vi "Process Data.vi"(7 "AdasLvTemplate in":refnum<class "AdasLvTemplate.lvclass">, 8 "error in":errorcluster, 11 "Node in":refnum<class "BLS Chiller Template.lvclass">) -> (0 "error out":errorcluster, 3 "Node out":refnum<class "BLS Chiller Template.lvclass">, 5 "AdasLvTemplate out":refnum<class "AdasLvTemplate.lvclass">)   [LabVIEW 2023, in "BLS Chiller Template.lvlib" / "BLS Chiller Template.lvclass"]
uses:
  BLS Chiller Template.lvclass
  <vilib>/ADAS Replay HIL/ADAS Plugin Utilities/AdasLvTemplate/AdasLvTemplate.lvclass
  BLS Chiller Template.lvclass/BLS Chiller Template.ctl
  bls-capabilities/src/Capabilities/High Level Capabilities/Chiller/Error Channels Write Array.vi
  bls-capabilities/src/Capabilities/High Level Capabilities/Chiller/Temperature Min Read Array.vi
  bls-capabilities/src/Capabilities/High Level Capabilities/Chiller/Temperature Max Read Array.vi
  bls-capabilities/src/Capabilities/High Level Capabilities/Chiller/Temperature Grad Read Array.vi
  bls-capabilities/src/Capabilities/High Level Capabilities/Chiller/Temperature Read Array.vi
  bls-capabilities/src/Capabilities/High Level Capabilities/Chiller/Pressure Min Read Array.vi
  bls-capabilities/src/Capabilities/High Level Capabilities/Chiller/Pressure Max Read Array.vi
  bls-capabilities/src/Capabilities/High Level Capabilities/Chiller/Pressure Grad Read Array.vi
  bls-capabilities/src/Capabilities/High Level Capabilities/Chiller/Pressure Read Array.vi
  bls-capabilities/src/Capabilities/High Level Capabilities/Chiller/Flow Max Read Array.vi
  bls-capabilities/src/Capabilities/High Level Capabilities/Chiller/Flow Min Read Array.vi
  bls-capabilities/src/Capabilities/High Level Capabilities/Chiller/Flow Read Array.vi
  bls-capabilities/src/Capabilities/High Level Capabilities/Chiller/Flow Grad Read Array.vi
  bls-capabilities/src/Capabilities/High Level Capabilities/Chiller/Temperature Write Array.vi
  bls-capabilities/src/Capabilities/High Level Capabilities/Chiller/Pressure Write Array.vi
  bls-capabilities/src/Capabilities/High Level Capabilities/Chiller/Flow Write Array.vi
  bls-capabilities/src/Capabilities/High Level Capabilities/Chiller/Chiller.lvclass
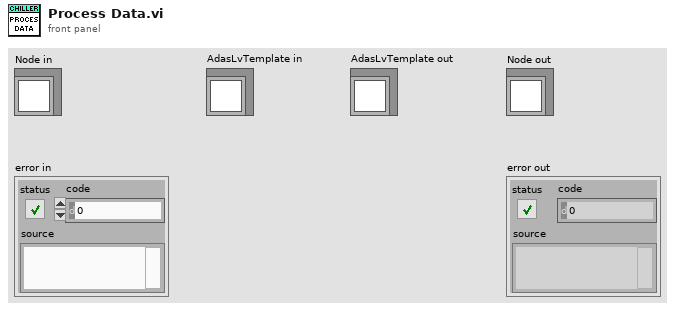
[diagram p1: front panel]
types:
  T1 = typedef "BLS Chiller Template.lvlib/BLS Chiller Template.lvclass/Configuration Params.ctl" = cluster{"Common":T2, "Amount of Channels":u32, "Address":string}
  T2 = typedef "Template Node.lvlib/Template Node.lvclass/Common Configuration Params.ctl" = cluster{"Iteration Interval (s)":dbl, "T0 (ns)":u64, "Priority":i32, "Processor":i32, "Wait in Ready State":bool}
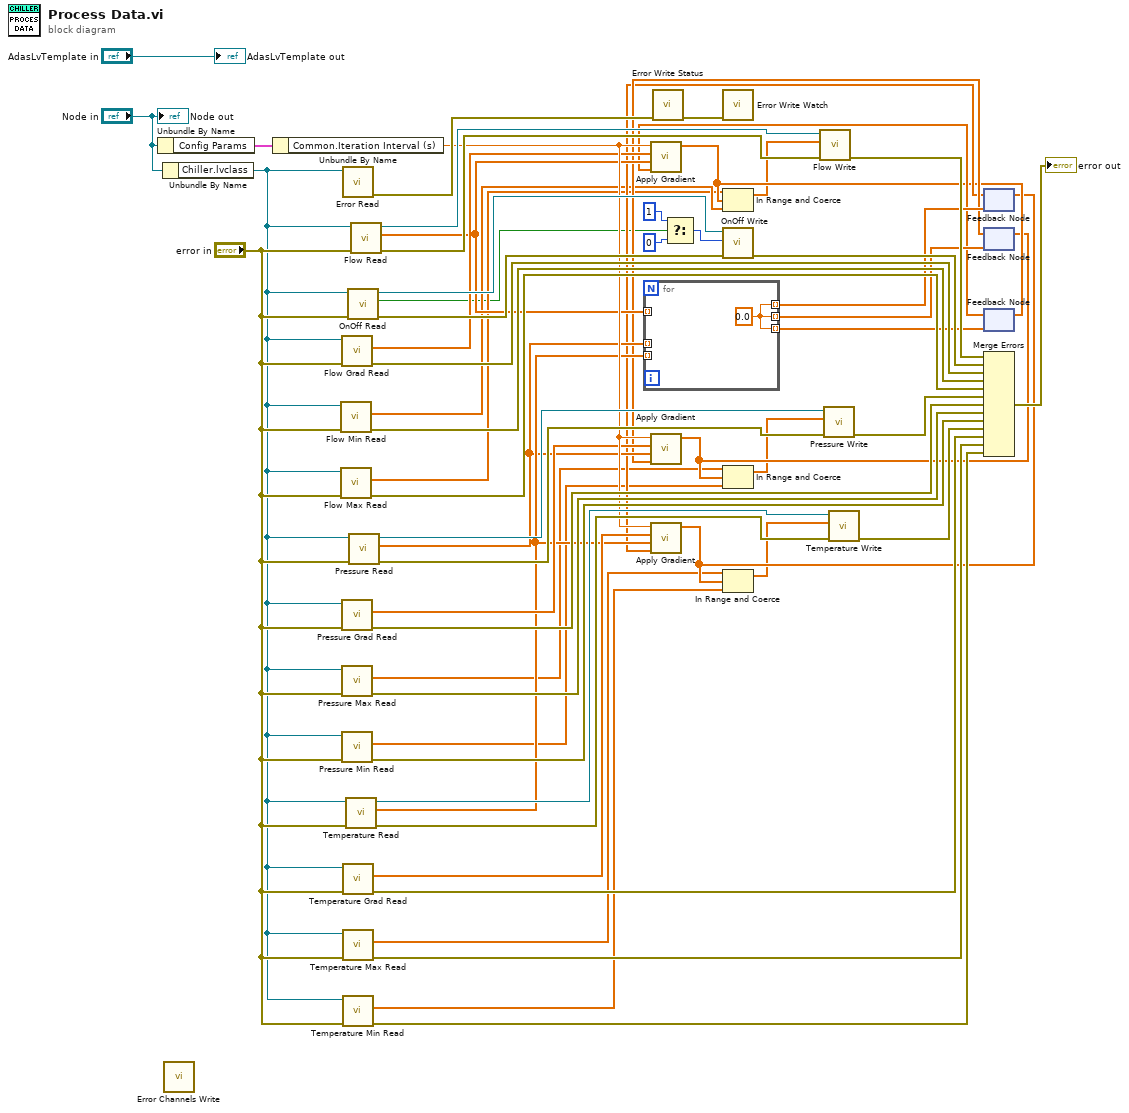
[diagram p0: block diagram]
diagram:
  n1 = Unbundle By Name("Node in") -> ("Config Params"=w30:T1)
  n2 = Unbundle By Name("Node in") -> ("Chiller.lvclass"=w33:refnum<class "Chiller.lvclass">)
  n3 = call-poly "Error Channels Write.vi"() -> ()  [unwired: 10 in, 2 out]
  n4 = Unbundle By Name(w30) -> ("Common.Iteration Interval (s)"=w29:dbl)
  n5 = call-poly "Flow Min Read.vi"("error in"="error in", "Chiller in"=w33) -> ("error out"=w43:errorcluster, "Flow Min SP"=w15:dbl[])  [unwired: 6 in, 2 out]
  n6 = call-poly "Flow Max Read.vi"("error in"="error in", "Chiller in"=w33) -> ("error out"=w42:errorcluster, "Flow Max SP"=w14:dbl[])  [unwired: 6 in, 2 out]
  n7 = call-poly "Flow Grad Read.vi"("error in"="error in", "Chiller in"=w33) -> ("error out"=w44:errorcluster, "Flow SP"=w28:dbl[])  [unwired: 6 in, 2 out]
  n8 = call-poly "Pressure Grad Read.vi"("error in"="error in", "Chiller in"=w33) -> ("error out"=w40:errorcluster, "Pressure SP"=w27:dbl[])  [unwired: 6 in, 2 out]
  n9 = call-poly "Pressure Max Read.vi"("error in"="error in", "Chiller in"=w33) -> ("error out"=w39:errorcluster, "Pressure Max SP"=w10:dbl[])  [unwired: 6 in, 2 out]
  n10 = call-poly "Pressure Min Read.vi"("error in"="error in", "Chiller in"=w33) -> ("error out"=w38:errorcluster, "Pressure Min SP"=w9:dbl[])  [unwired: 6 in, 2 out]
  n11 = call "Error Read.vi"("Chiller in"=w33) -> ("error out"=w53:errorcluster)  [unwired: 7 in, 3 out]
  n12 = call-poly "Temperature Grad Read.vi"("error in"="error in", "Chiller in"=w33) -> ("error out"=w36:errorcluster, "Temperature SP"=w26:dbl[])  [unwired: 6 in, 2 out]
  n13 = call-poly "Temperature Max Read.vi"("error in"="error in", "Chiller in"=w33) -> ("error out"=w35:errorcluster, "Temperature Max SP"=w6:dbl[])  [unwired: 6 in, 2 out]
  n14 = call-poly "Temperature Min Read.vi"("error in"="error in", "Chiller in"=w33) -> ("error out"=w34:errorcluster, "Temperature Min SP"=w7:dbl[])  [unwired: 6 in, 2 out]
  n15 = call-poly "Temperature Read.vi"("error in"="error in", "Chiller in"=w33) -> ("error out"=w46:errorcluster, "Temperature SP"=w22:dbl[], "Chiller out"=w45:refnum<class "Chiller.lvclass">)  [unwired: 6 in, 1 out]
  n16 = call "OnOff Read.vi"("error in"="error in", "Chiller in"=w33) -> ("error out"=w51:errorcluster, "OnOff ACT"=w2:bool, "Chiller out"=w50:refnum<class "Chiller.lvclass">)  [unwired: 6 in, 1 out]
  n17 = call-poly "Pressure Read.vi"("error in"="error in", "Chiller in"=w33) -> ("error out"=w48:errorcluster, "Pressure SP"=w21:dbl[], "Chiller out"=w49:refnum<class "Chiller.lvclass">)  [unwired: 6 in, 1 out]
  n18 = call-poly "Flow Read.vi"("error in"="error in", "Chiller in"=w33) -> ("error out"=w55:errorcluster, "Flow SP"=w20:dbl[], "Chiller out"=w54:refnum<class "Chiller.lvclass">)  [unwired: 6 in, 1 out]
  n19 = for {
    tunnel: [w59] -> w25 mode=indexing
    tunnel: [w59] -> w24 mode=indexing
    tunnel: w21 -> [_] mode=indexing
    tunnel: [w59] -> w23 mode=indexing
    tunnel: w22 -> [_] mode=indexing
    tunnel: w20 -> [_] mode=indexing
    w59 = 0.0 ("Current Setpoint")
  }
  n20 = call "Error Write Status.vi"("error in"=w53) -> ("error out"=w52:errorcluster)  [unwired: 9 in, 1 out]
  n21 = Select(t=1, s=w2, f=0) -> (s? t:f=w1:i32)
  n22 = call "Error Write Watch.vi"("error in"=w52) -> ()  [unwired: 9 in, 2 out]
  n23 = call "OnOff Write.vi"("error in"=w51, "OnOff STS"=w1, "Chiller in"=w50) -> ("error out"=w58:errorcluster)  [unwired: 7 in, 1 out]
  n24 = feedback #1(w23) -> (w17:dbl[])
  n25 = call "Apply Gradient.vi"("Reminder"=w17, "Setpoint"=w22, "Gradient"=w26, "Iteration Interval"=w29) -> ("Array"=w8:dbl[])  [unwired: 7 in]
  n26 = In Range and Coerce(upper limit=w6, x=w8, lower limit=w7) -> (coerced(x)=w5:dbl[])  [unwired: 1 out]
  n27 = call-poly "Temperature Write.vi"("error in"=w46, "Temperature AV"=w5, "Chiller in"=w45) -> ("error out"=w37:errorcluster)  [unwired: 7 in, 1 out]
  n28 = feedback-in #1(w8) -> ()
  n29 = feedback #2(w24) -> (w18:dbl[])
  n30 = call "Apply Gradient.vi"("Reminder"=w18, "Setpoint"=w21, "Gradient"=w27, "Iteration Interval"=w29) -> ("Array"=w12:dbl[])  [unwired: 7 in]
  n31 = In Range and Coerce(upper limit=w10, x=w12, lower limit=w9) -> (coerced(x)=w11:dbl[])  [unwired: 1 out]
  n32 = call-poly "Pressure Write.vi"("error in"=w48, "Pressure AV"=w11, "Chiller in"=w49) -> ("error out"=w41:errorcluster)  [unwired: 7 in, 1 out]
  n33 = feedback-in #2(w12) -> ()
  n34 = feedback #3(w25) -> (w19:dbl[])
  n35 = call "Apply Gradient.vi"("Reminder"=w19, "Setpoint"=w20, "Gradient"=w28, "Iteration Interval"=w29) -> ("Array"=w16:dbl[])  [unwired: 7 in]
  n36 = In Range and Coerce(upper limit=w14, x=w16, lower limit=w15) -> (coerced(x)=w13:dbl[])  [unwired: 1 out]
  n37 = call-poly "Flow Write.vi"("error in"=w55, "Flow AV"=w13, "Chiller in"=w54) -> ("error out"=w32:errorcluster)  [unwired: 7 in, 1 out]
  n38 = feedback-in #3(w16) -> ()
  n39 = Merge Errors(w32, w58, w44, w43, w42, w41, w40, w39, w38, w37, w36, w35, w34) -> (→"error out":errorcluster)
  "Node out" <- "Node in"
  "AdasLvTemplate out" <- "AdasLvTemplate in"
